vi "Read Server Internal UEs.vi"(8 "error in (no error)":errorcluster, 11 "gRPC service in":refnum<class "Session.lvclass">) -> (0 "error out":errorcluster, 2 "Server Internal UEs":T1, 3 "gRPC service out":refnum<class "Session.lvclass">)   [LabVIEW 2019, in "Generated_server.lvlib" / "Session.lvclass"]
uses:
  Session.lvclass
  typeDefs/Server Internal UEs.ctl
  typeDefs/Server Internal Message.ctl
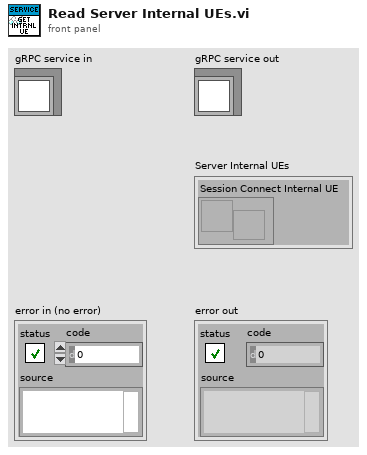
[diagram p1: front panel]
types:
  T1 = typedef "Generated_server.lvlib/Session.lvclass/Server Internal UEs.ctl" = cluster{"Session Connect Internal UE":refnum<user-event>}
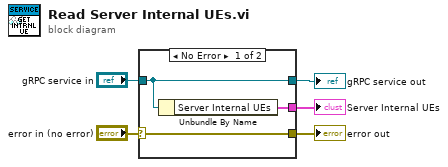
[diagram p0: block diagram]
diagram:
  n1 = case shown="No Error" "error in (no error)" {
    selector: "error in (no error)" -> [w8 w9]
    tunnel: [w8 w9] -> w4
    tunnel: [w7 w10] -> w2
    tunnel: "gRPC service in" -> [w7 w10]
    tunnel: [w6 _] -> w1
    frame No Error {
      n2 = Unbundle By Name(w7) -> ("Server Internal UEs"=w6:T1)
    }
    frame Error {
    }
  }
  "error out" <- w4
  "gRPC service out" <- w2
  "Server Internal UEs" <- w1
